vi "Create ListImp_Populated.vi"(5 "ListImp_Populated in":refnum<class "ListImp_Populated.lvclass">, 8 "error in (no error)":errorcluster, 10 "Initial List":i32[](array[numeric]), 11 "ListImp":refnum<class "ListImp.lvclass">) -> (0 "error out":errorcluster, 3 "ListImp_Populated out":refnum<class "ListImp_Populated.lvclass">)   [LabVIEW 2013, in "ListImp_Populated.lvclass"]
uses:
  ListImp_Populated.lvclass
  source/LapDog.Collections.Lists/ListImp/ListImp.lvclass
  ListImp_Populated.lvclass/ListImp_Populated.ctl
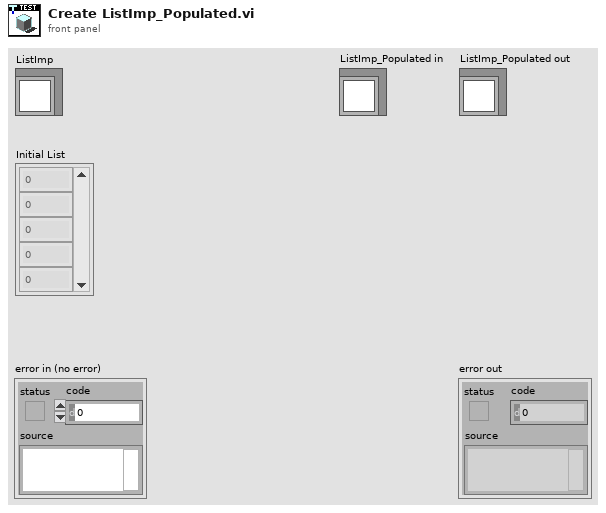
[diagram p1: front panel]
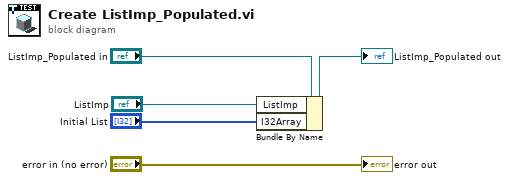
[diagram p0: block diagram]
diagram:
  n1 = Bundle By Name(cluster="ListImp_Populated in", "ListImp"="ListImp", "I32Array"="Initial List") -> (→"ListImp_Populated out":refnum<class "ListImp_Populated.lvclass">)
  "error out" <- "error in (no error)"
